vi "Ignore Errors Before.vi"(8 "error in (no error)":errorcluster) -> (0 "error out":errorcluster)   [LabVIEW 2014, in "UI_ProgressDlg.lvlib" / "UI_ProgressDlg.lvclass"]
uses:
  UI_ProgressDlg.lvclass
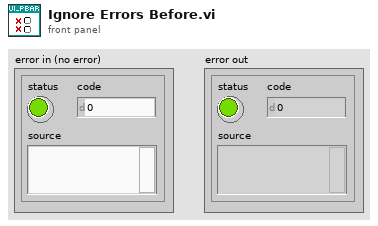
[diagram p1: front panel]
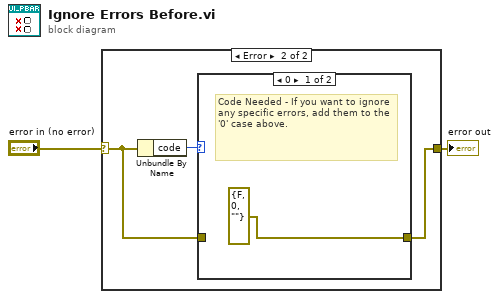
[diagram p0: block diagram]
diagram:
  n1 = case shown="Error" "error in (no error)" {
    selector: "error in (no error)" -> [w3 w5]
    tunnel: [w3 w4] -> w2
    frame No Error {
    }
    frame Error {
      n2 = Unbundle By Name(w5) -> ("code"=w6:i32)
      n3 = case shown="0" w6 {
        tunnel: [errorcluster {"status"=FALSE, "code"=0, "source"=""} ("error constant") w8] -> w4
        tunnel: w5 -> [_ w8]
        frame 0 {
          # "Code Needed - If you want to ignore any specific errors, add them to the '0' case above."
        }
        frame Default {
        }
      }
    }
  }
  "error out" <- w2
